vi "example_dynamically_invoking - master.vi"() -> ()   [LabVIEW 2012]
doc: "This example VI (the Master) demonstrates the capabilities of controlling a dynamically loaded VI that solely acts as a controller mechanism for an attached device. This might serve useful for a plug-in type architecture where one might develop against an interface for motor / motion control.\n\nTo operate, simply 'start' this VI and it should automatically invoke methods for (1) selecting the attached device, (2) instantiating the selected device and (3) controlling simple functions such as jogging forward and backward. Again, all motor control happens in the dynamically loaded (Slave) VI (example_dynamically_invoking - slave.vi). This Slave VI must exist in the same directory as the Master.\n\nProduced By:\n\nChristopher Lemieux\nKod Integrations, LLC\n4835 Marianne Drive\nMount Airy, MD 21771\nhttp://www.kodintegrations.com\nemail: clemieux@kodintegrations.com\nphone: (240) 687-1288"
uses:
  controls/example_dynamically_invoking - master_action_item.ctl
  controls/example_dynamically_invoking - master_actions.ctl
  controls/example_dynamically_invoking - slave_actions.ctl
panel:
  in  "terminate":bool
  in  "jog_neg":bool caption="Jog (-)"
  in  "jog_pos":bool caption="Jog (+)"
  in  "slow_stop":bool caption="Stop Slowly"
  out "slave_err (out)":errorcluster
  out "error out":errorcluster
  in  "error in (no error)":errorcluster
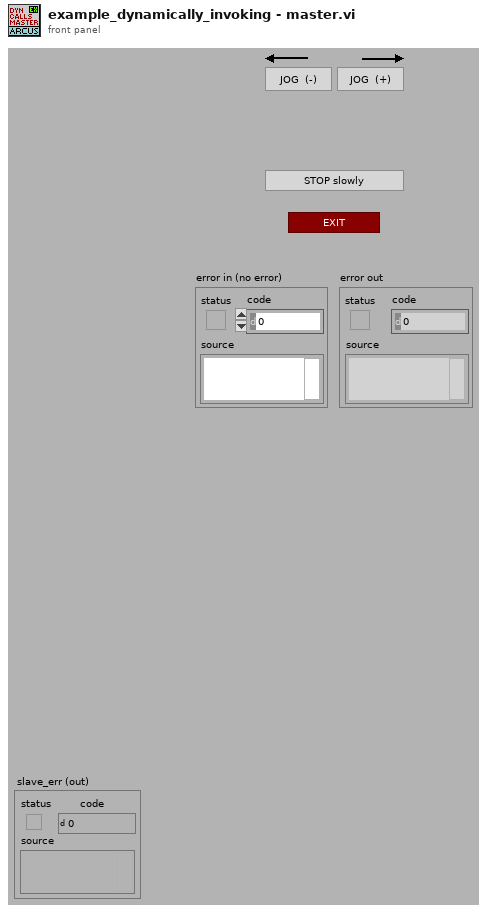
[diagram p1: front panel]
types:
  T1 = typedef "example_dynamically_invoking - master_action_item.ctl" = cluster{"actions":T2, "data":variant}
  T2 = typedef "example_dynamically_invoking - master_actions.ctl" = enum16{"exit", "getError", "initialize", "processEvents", "runSlave", "setSlaveAction"}
  T3 = typedef "example_dynamically_invoking - slave_actions.ctl" = enum16{"exit", "initialize", "jogConstNeg", "jogConstPos", "stopSlowly"}
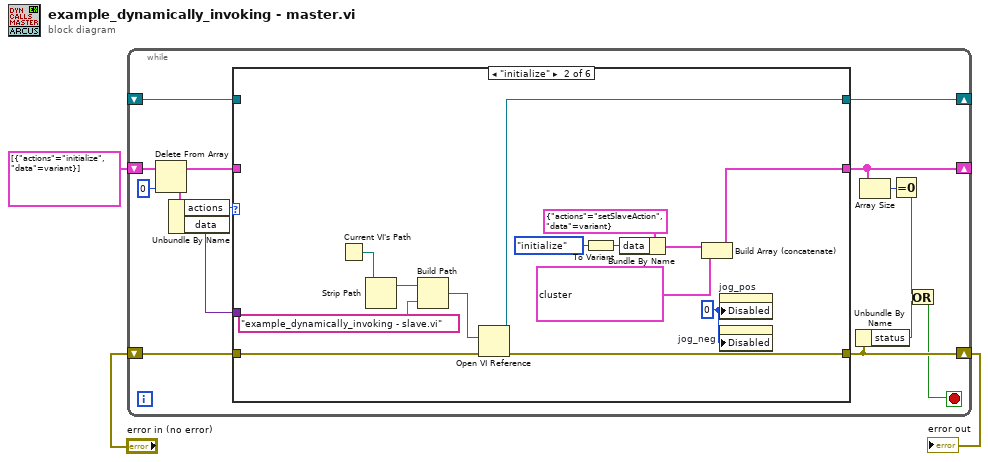
[diagram p0: block diagram]
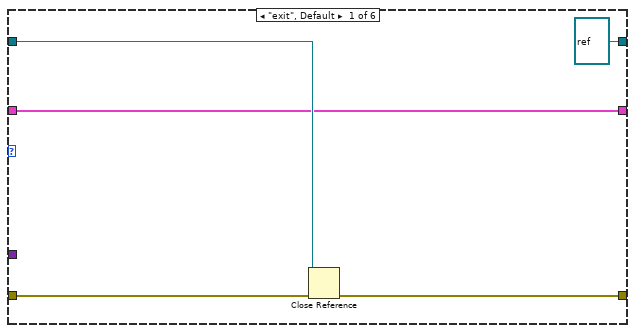
[diagram p2: hidden frame]
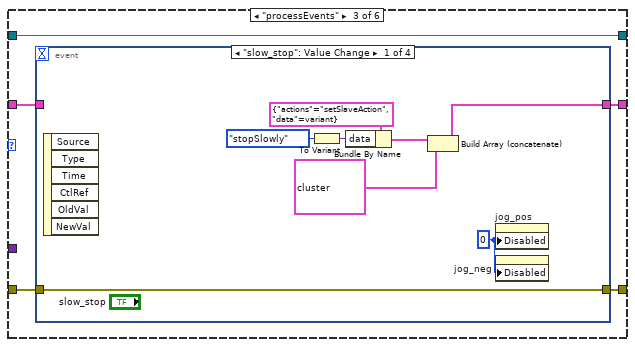
[diagram p3: hidden frame]
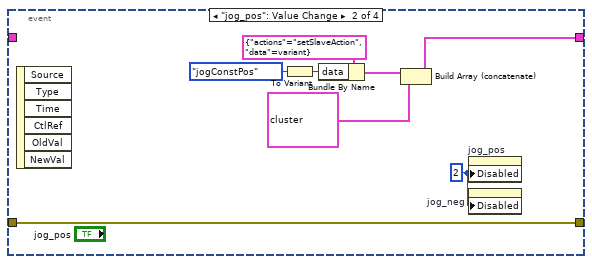
[diagram p4: hidden frame]
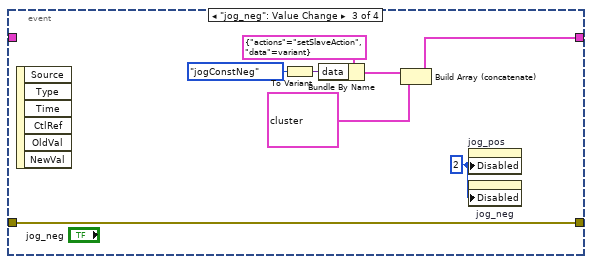
[diagram p5: hidden frame]
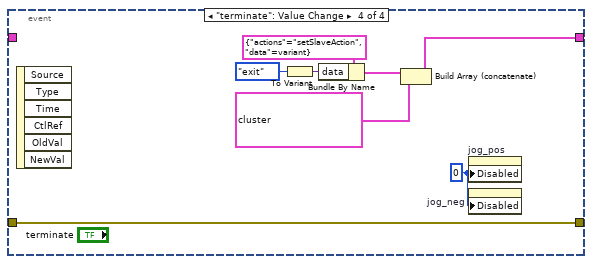
[diagram p6: hidden frame]
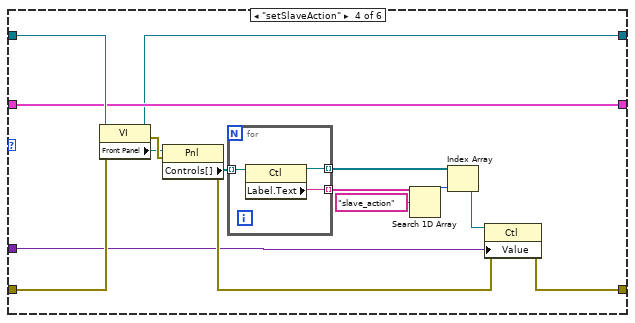
[diagram p7: hidden frame]
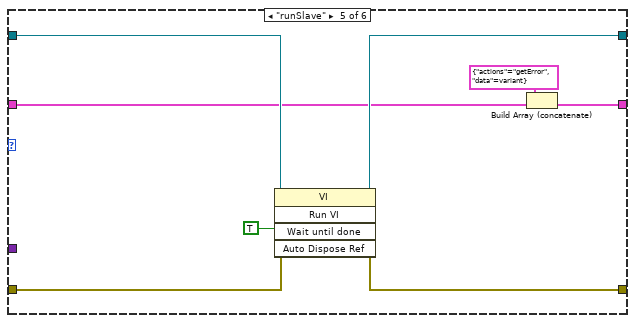
[diagram p8: hidden frame]
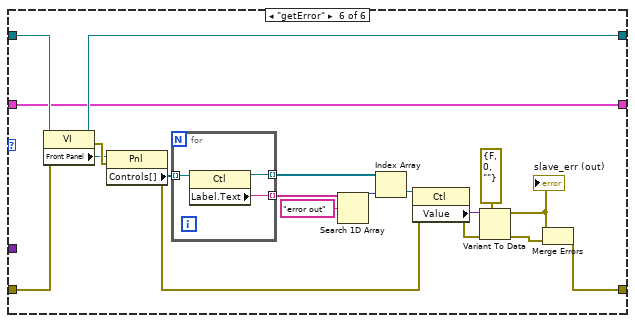
[diagram p9: hidden frame]
diagram:
  n1 = while {
    shift-right: [w12] -> _
    shift-left: T1[] [{"actions"=enum."initialize", "data"=variant}] -> [w18]
    shift-right: [w10] -> w1
    shift-left: "error in (no error)" -> [w15]
    shift-right: [w14] -> _
    shift-left: _ -> [w13]
    stop <- w7 stop-if-true
    n2 = Delete From Array(array=w18, index=0) -> (deleted portion=w6:T1, array with subset deleted=w16:T1[])  [unwired: 1 in]
    n3 = Unbundle By Name(w6) -> ("actions"=w5:T2, "data"=w4:variant)
    n4 = case shown="\"initialize\"" w5 {
      tunnel: w16 -> [w19 _ w41 w76 w94 w104]
      tunnel: w15 -> [w23 w37 w40 w79 w97 w107]
      tunnel: [w22 w31 w39 w77 w96 w101] -> w10
      tunnel: [refnum<vi> refnum w32 w42 w75 w99 w108] -> w14
      tunnel: w13 -> [w21 _ w42 w80 w100 w109]
      tunnel: [w19 w25 w38 w76 w93 w104] -> w12
      tunnel: w4 -> [_ _ _ w78 _ _]
      frame "exit", Default {
        n5 = Close Reference(reference=w21, error in (no error)=w23) -> (error out=w22:errorcluster)
      }
      frame "initialize" {
        w24 = u8 0 ("Disabled")
        n6 = Current VI's Path() -> (path=w36:path)
        n7 = Strip Path(path=w36) -> (stripped path=w35:path)  [unwired: 1 out]
        n8 = Build Path(base path=w35, name or relative path="example_dynamically_invoking - slave.vi") -> (appended path=w33:path)
        n9 = Open VI Reference(vi path=w33, error in (no error)=w37) -> (vi reference=w32:refnum<vi>, error out=w31:errorcluster)  [unwired: 4 in]
        n10 = To Variant(anything=example_dynamically_invoking_-_slave_actions."initialize" ("slave_action")) -> (Variant=w29:variant)
        n11 = Bundle By Name(cluster=T1 {"actions"=enum."setSlaveAction", "data"=variant} ("action_item"), "data"=w29) -> (w28:T1)
        n12 = Build Array (concatenate)(w28, T1[] [{"actions"=enum."runSlave", "data"=variant}, {"actions"=enum."processEvents", "data"=variant}]) -> (w25:T1[])
        n13 = property on="jog_pos" class="Bool"("Disabled"=w24) -> ()  [unwired: 2 in, 2 out]
        n14 = property on="jog_neg" class="Bool"("Disabled"=w24) -> ()  [unwired: 2 in, 2 out]
      }
      frame "processEvents" {
        n15 = event shown="[0] \"slow_stop\": Value Change" {
          selector: _ -> [_ _ _ _]
          dyn-events: _ -> [_ _ _ _]
          timeout: _ -> [_ _ _ _]
          tunnel: w41 -> [_ _ _ _]
          tunnel: w40 -> [w50 w58 w66 w74]
          tunnel: [w50 w58 w66 w74] -> w39
          tunnel: [w45 w53 w61 w69] -> w38
          event "slow_stop": Value Change {
            w43 = u8 0 ("Disabled")
            n16 = event-data() -> ()  [unwired: 1 in, 6 out]
            n17 = To Variant(anything=example_dynamically_invoking_-_slave_actions."stopSlowly" ("slave_action")) -> (Variant=w48:variant)
            n18 = Bundle By Name(cluster=T1 {"actions"=enum."setSlaveAction", "data"=variant} ("action_item"), "data"=w48) -> (w47:T1)
            n19 = Build Array (concatenate)(w47, T1[] [{"actions"=enum."runSlave", "data"=variant}, {"actions"=enum."processEvents", "data"=variant}]) -> (w45:T1[])
            n20 = property on="jog_pos" class="Bool"("Disabled"=w43) -> ()  [unwired: 2 in, 2 out]
            n21 = property on="jog_neg" class="Bool"("Disabled"=w43) -> ()  [unwired: 2 in, 2 out]
          }
          event "jog_pos": Value Change {
            w51 = u8 2 ("Disabled")
            n22 = event-data() -> ()  [unwired: 1 in, 6 out]
            n23 = To Variant(anything=example_dynamically_invoking_-_slave_actions."jogConstPos" ("slave_action")) -> (Variant=w56:variant)
            n24 = Bundle By Name(cluster=T1 {"actions"=enum."setSlaveAction", "data"=variant} ("action_item"), "data"=w56) -> (w55:T1)
            n25 = Build Array (concatenate)(w55, T1[] [{"actions"=enum."runSlave", "data"=variant}, {"actions"=enum."processEvents", "data"=variant}]) -> (w53:T1[])
            n26 = property on="jog_pos" class="Bool"("Disabled"=w51) -> ()  [unwired: 2 in, 2 out]
            n27 = property on="jog_neg" class="Bool"("Disabled"=w51) -> ()  [unwired: 2 in, 2 out]
          }
          event "jog_neg": Value Change {
            w59 = u8 2 ("Disabled")
            n28 = event-data() -> ()  [unwired: 1 in, 6 out]
            n29 = To Variant(anything=example_dynamically_invoking_-_slave_actions."jogConstNeg" ("slave_action")) -> (Variant=w64:variant)
            n30 = Bundle By Name(cluster=T1 {"actions"=enum."setSlaveAction", "data"=variant} ("action_item"), "data"=w64) -> (w63:T1)
            n31 = Build Array (concatenate)(w63, T1[] [{"actions"=enum."runSlave", "data"=variant}, {"actions"=enum."processEvents", "data"=variant}]) -> (w61:T1[])
            n32 = property on="jog_pos" class="Bool"("Disabled"=w59) -> ()  [unwired: 2 in, 2 out]
            n33 = property on="jog_neg" class="Bool"("Disabled"=w59) -> ()  [unwired: 2 in, 2 out]
          }
          event "terminate": Value Change {
            w67 = u8 0 ("Disabled")
            n34 = event-data() -> ()  [unwired: 1 in, 6 out]
            n35 = To Variant(anything=example_dynamically_invoking_-_slave_actions."exit" ("slave_action")) -> (Variant=w72:variant)
            n36 = Bundle By Name(cluster=T1 {"actions"=enum."setSlaveAction", "data"=variant} ("action_item"), "data"=w72) -> (w71:T1)
            n37 = Build Array (concatenate)(w71, T1[] [{"actions"=enum."runSlave", "data"=variant}, {"actions"=enum."exit", "data"=variant}]) -> (w69:T1[])
            n38 = property on="jog_pos" class="Bool"("Disabled"=w67) -> ()  [unwired: 2 in, 2 out]
            n39 = property on="jog_neg" class="Bool"("Disabled"=w67) -> ()  [unwired: 2 in, 2 out]
          }
        }
      }
      frame "setSlaveAction" {
        n40 = property class="VI"(reference=w80, error in=w79) -> (reference out=w75:refnum<vi>, error out=w83:errorcluster, "Front Panel"=w82:refnum<vi>)
        n41 = property class="Pnl"(reference=w82, error in=w83) -> (error out=w81:errorcluster, "Controls[]"=w84:refnum<vi>[])  [unwired: 1 out]
        n42 = for {
          tunnel: w84 -> [w92] mode=indexing
          tunnel: [w91] -> w85 mode=indexing
          tunnel: [w90] -> w87 mode=indexing
          n43 = property class="Ctl"(reference=w92) -> (reference out=w90:refnum<vi>, "Label.Text"=w91:string)  [unwired: 1 in, 1 out]
        }
        n44 = Search 1D Array(1D array=w85, element="slave_action") -> (index of element=w88:i32)  [unwired: 1 in]
        n45 = Index Array(array=w87, index=w88) -> (element=w89:refnum<vi>)
        n46 = property class="Ctl"(reference=w89, error in=w81, "Value"=w78) -> (error out=w77:errorcluster)  [unwired: 1 out]
      }
      frame "runSlave" {
        n47 = invoke class="VI" method="Run VI"(reference=w100, error in=w97, "Wait until done"=TRUE) -> (reference out=w99:refnum<vi>, error out=w96:errorcluster)  [unwired: 2 in, 3 out]
        n48 = Build Array (concatenate)(T1 {"actions"=enum."getError", "data"=variant} ("action_item"), w94) -> (w93:T1[])
      }
      frame "getError" {
        n49 = property class="VI"(reference=w109, error in=w107) -> (reference out=w108:refnum<vi>, error out=w111:errorcluster, "Front Panel"=w110:refnum<vi>)
        n50 = property class="Pnl"(reference=w110, error in=w111) -> (error out=w106:errorcluster, "Controls[]"=w112:refnum<vi>[])  [unwired: 1 out]
        n51 = for {
          tunnel: w112 -> [w122] mode=indexing
          tunnel: [w121] -> w113 mode=indexing
          tunnel: [w120] -> w115 mode=indexing
          n52 = property class="Ctl"(reference=w122) -> (reference out=w120:refnum<vi>, "Label.Text"=w121:string)  [unwired: 1 in, 1 out]
        }
        n53 = Search 1D Array(1D array=w113, element="error out") -> (index of element=w116:i32)  [unwired: 1 in]
        n54 = Index Array(array=w115, index=w116) -> (element=w117:refnum<vi>)
        n55 = property class="Ctl"(reference=w117, error in=w106) -> (error out=w105:errorcluster, "Value"=w118:variant)  [unwired: 1 out]
        n56 = Variant To Data(error in=w105, type=errorcluster {"status"=FALSE, "code"=0, "source"=""} ("error out"), Variant=w118) -> (data=w103:errorcluster, error out=w102:errorcluster)
        "slave_err (out)" <- w103
        n57 = Merge Errors(w103, w102) -> (w101:errorcluster)
      }
    }
    n58 = Unbundle By Name(w10) -> ("status"=w8:bool)
    n59 = Array Size(array=w12) -> (size(s)=w11:i32)
    n60 = Equal To 0?(x=w11) -> (x = 0?=w9:bool)
    n61 = Or(x=w9, y=w8) -> (x .or. y?=w7:bool)
  }
  "error out" <- w1
